vi "Read Emergency Status.vi"(11 "Emergency Status Msg in":refnum<class "Emergency Status Msg.lvclass">) -> (2 "Content":string, 3 "Emergency Status Msg out":refnum<class "Emergency Status Msg.lvclass">)   [LabVIEW 2015, in "SCADA Core.lvlib" / "Emergency Status Msg.lvclass"]
uses:
  Emergency Status Msg.lvclass
  Emergency Status Msg.lvclass/Emergency Status Msg.ctl
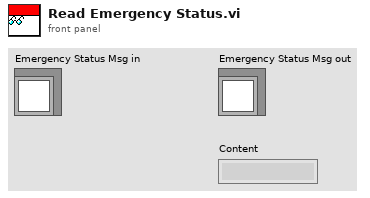
[diagram p1: front panel]
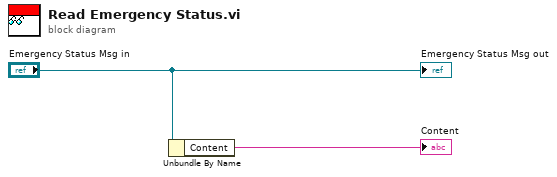
[diagram p0: block diagram]
diagram:
  n1 = Unbundle By Name("Emergency Status Msg in") -> ("Content"=→"Content":string)
  "Emergency Status Msg out" <- "Emergency Status Msg in"
